vi "DevB.Send Message I32.vi"(8 "error in (no error)":errorcluster, 9 "data":i32, 10 "Message":T1, 11 "DevB.Message queue in":refnum<queue>) -> (0 "error out":errorcluster, 3 "DevB.Message queue out":refnum<queue>)   [LabVIEW 2018]
uses:
  typedefs/DevB.Message type.ctl
  typedefs/DevB.Message.ctl
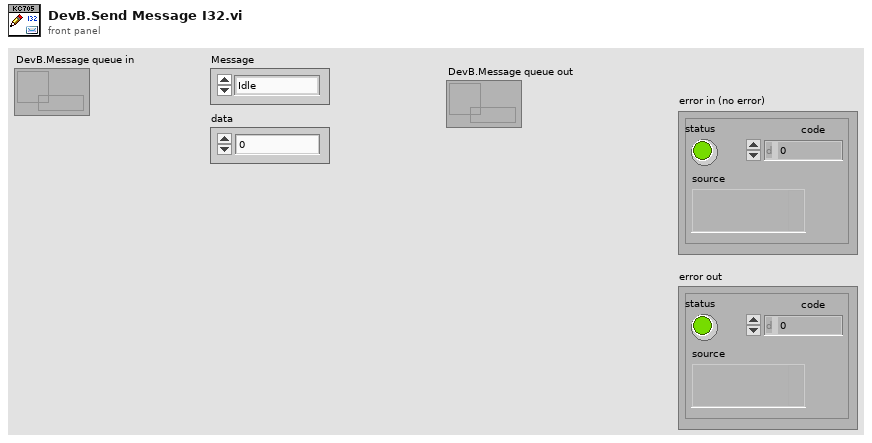
[diagram p1: front panel]
types:
  T1 = typedef "DevB.Message type.ctl" = enum16{"Idle", "Set Duration", "Set Frequency", "Set Phase", "Set Delay", "on/off", "check status"}
  T2 = typedef "DevB.Message.ctl" = cluster{"type":T1, "data":variant}
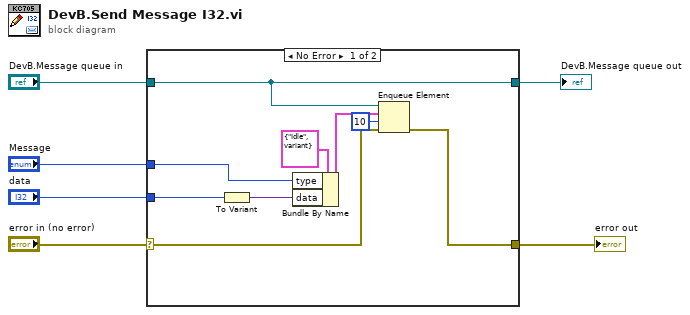
[diagram p0: block diagram]
diagram:
  n1 = case shown="No Error" "error in (no error)" {
    selector: "error in (no error)" -> [w10 w17]
    tunnel: "data" -> [w13 _]
    tunnel: "Message" -> [w11 _]
    tunnel: [w9 w17] -> w3
    tunnel: "DevB.Message queue in" -> [w7 w16]
    tunnel: [w7 w16] -> w1
    frame No Error {
      n2 = To Variant(anything=w13) -> (Variant=w12:variant)
      n3 = Bundle By Name(cluster=T2 {"type"=enum."Idle", "data"=variant} ("element"), "type"=w11, "data"=w12) -> (w14:T2)
      n4 = Enqueue Element(queue=w7, element=w14, timeout in ms (-1)=10, error in (no error)=w10) -> (error out=w9:errorcluster)  [unwired: 2 out]
    }
    frame Error {
    }
  }
  "error out" <- w3
  "DevB.Message queue out" <- w1
